vi "Idle_Insert.vi"(4 "Serial No":i32, 8 "error in (no error)":errorcluster, 11 "Ref in":T1={"MS SQL Connection"=refnum, "UDL File"=path "", "Time"="", "DCODE"="", "WIP+1"=0, "MC No?"=0, "POKAYOKE?"=FALSE, "Expected Result"="", "Result [Status]"="", "Clock"=0.0, "RFID"="", "WIP Queue"=refnum, "TS Parameter"={"ProfitCenterCode"="", "LineCode"="", "WorkOrderNumber"="", "Model"="", "Model_with_Prefix"="", "VendorCode"="", "SetParameterDateCode"="", "PokaYoke"=0, "Target"=1, "Live_DateCode"="", "CustomerPartNumber"="", "Hand"="", "sBarcode"=FALSE, "FCA"=0, "Ent_Stamp"=timestamp(0 s since 1904-01-01), "STS_CD"=0.0}, "Data_Queue"=[], "RFID Serial No."=""} {"TS Parameter"."FCA" format="%01d"; "TS Parameter"."Target" min=1 max=100000; "TS Parameter"."PokaYoke" min=0 max=1}) -> (0 "error out":errorcluster, 2 "Message":picture, 3 "Ref Out":T1={"MS SQL Connection"=refnum, "UDL File"=path "", "Time"="", "DCODE"="", "WIP+1"=0, "MC No?"=0, "POKAYOKE?"=FALSE, "Expected Result"="", "Result [Status]"="", "Clock"=0.0, "RFID"="", "WIP Queue"=refnum, "TS Parameter"={"ProfitCenterCode"="", "LineCode"="", "WorkOrderNumber"="", "Model"="", "Model_with_Prefix"="", "VendorCode"="", "SetParameterDateCode"="", "PokaYoke"=0, "Target"=1, "Live_DateCode"="", "CustomerPartNumber"="", "Hand"="", "sBarcode"=FALSE, "FCA"=0, "Ent_Stamp"=timestamp(0 s since 1904-01-01), "STS_CD"=0.0}, "Data_Queue"=[], "RFID Serial No."=""} {"TS Parameter"."FCA" format="%01d"; "TS Parameter"."Target" min=1 max=100000; "TS Parameter"."PokaYoke" min=0 max=1})   [LabVIEW 2020]
uses:
  Controls/TD SQL.ctl
  <vilib>/addons/database/Connection.llb/Conn ObjectReference.ctl
  Controls/WIP_State.ctl
  Controls/TS_Parameter.ctl
  Controls/Msg_Type.ctl
  MS SQL/MS_Global.vi
  <vilib>/addons/database/NI_Database_API.lvlib
panel:
  out "resulting string":string
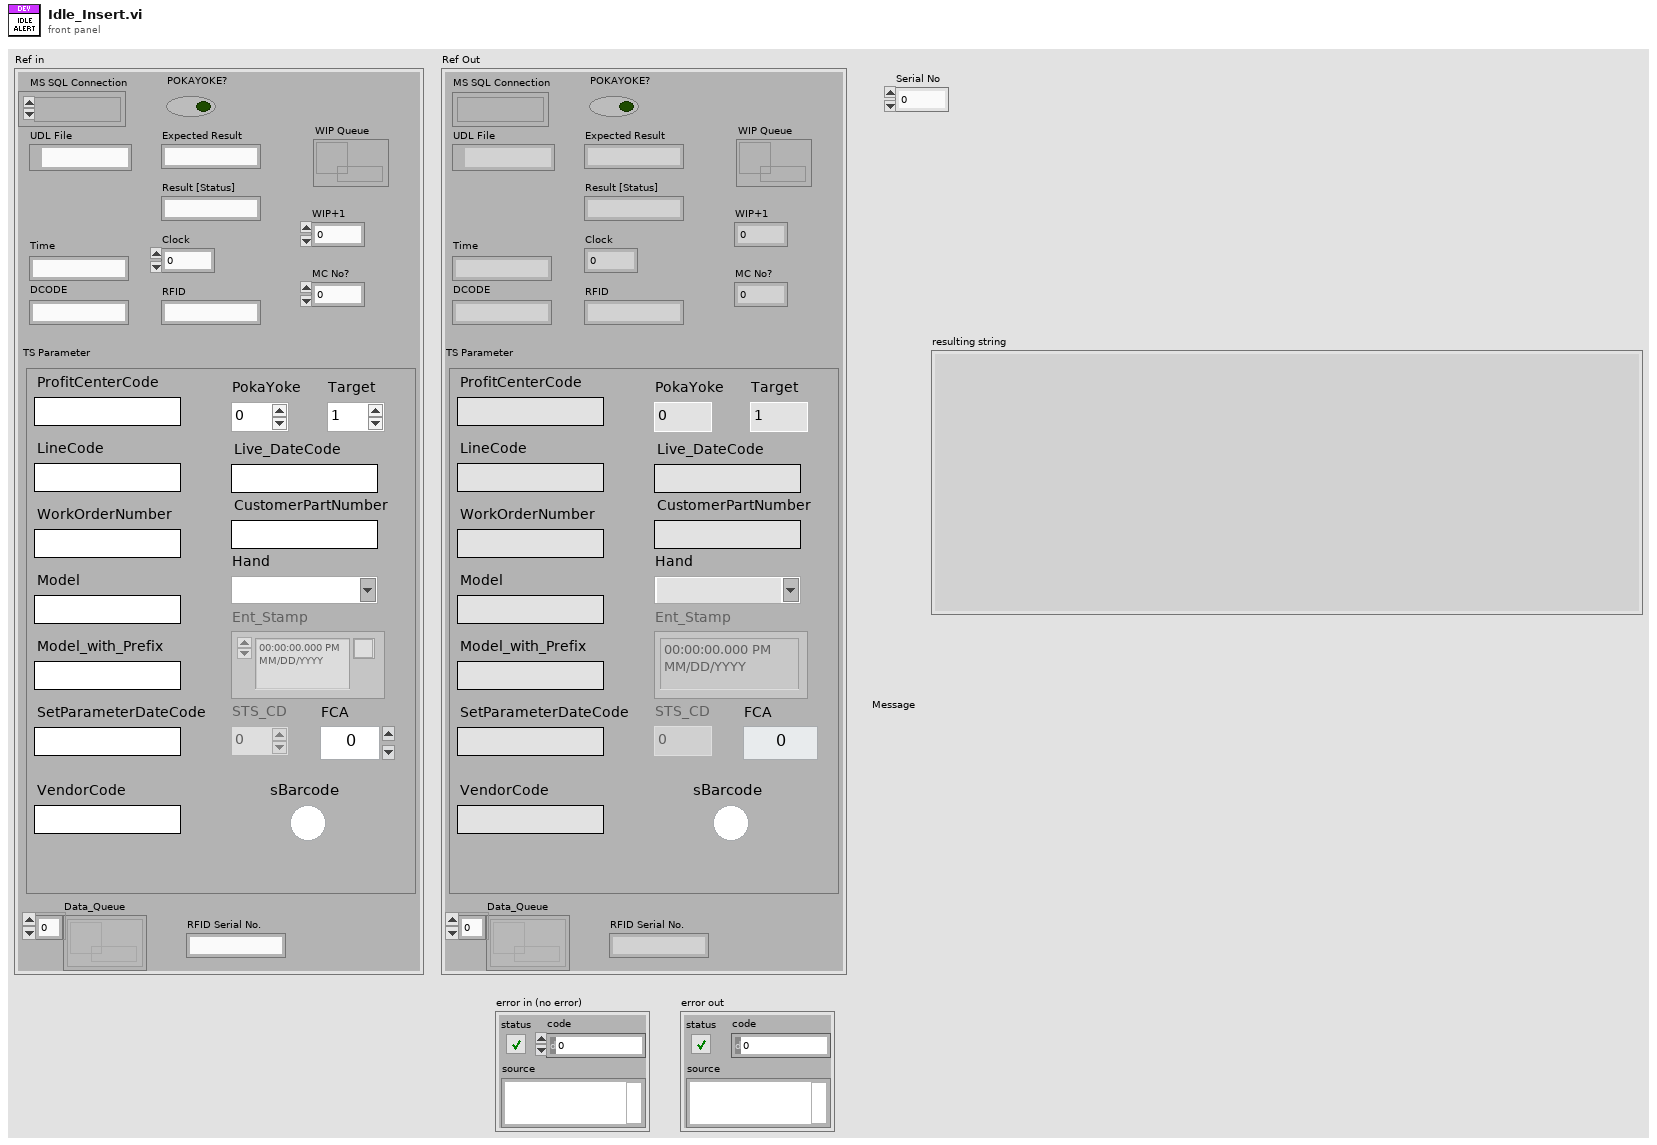
[diagram p1: front panel]
types:
  T1 = typedef "TD SQL.ctl" = cluster{"MS SQL Connection":T2, "UDL File":path, "Time":string, "DCODE":string, "WIP+1":i64, "MC No?":i32, "POKAYOKE?":bool, "Expected Result":string, "Result [Status]":string, "Clock":dbl, "RFID":string, "WIP Queue":refnum<queue>, "TS Parameter":T3, "Data_Queue":refnum<queue>[], "RFID Serial No.":string}
  T2 = typedef "NI_Database_API.lvlib/Conn ObjectReference.ctl" = refnum<k1>
  T3 = typedef "TS_Parameter.ctl" = cluster{"ProfitCenterCode":string, "LineCode":string, "WorkOrderNumber":string, "Model":string, "Model_with_Prefix":string, "VendorCode":string, "SetParameterDateCode":string, "PokaYoke":i32, "Target":i32, "Live_DateCode":string, "CustomerPartNumber":string, "Hand":string, "sBarcode":bool, "FCA":i32, "Ent_Stamp":timestamp, "STS_CD":dbl}
  T4 = typedef "Msg_Type.ctl" = enum16{"Normal", "Pass", "Fail", "Fault", "User", "Bypass", "Fail Save"}
  T5 = typedef "Idle_Timer.ctl" = cluster{"OP10":T6, "OP20":T6, "OP30":T6, "OP40":T6, "OP50":T6, "OP60":T6}
  T6 = typedef "Idle_Timer_disp.ctl" = dbl
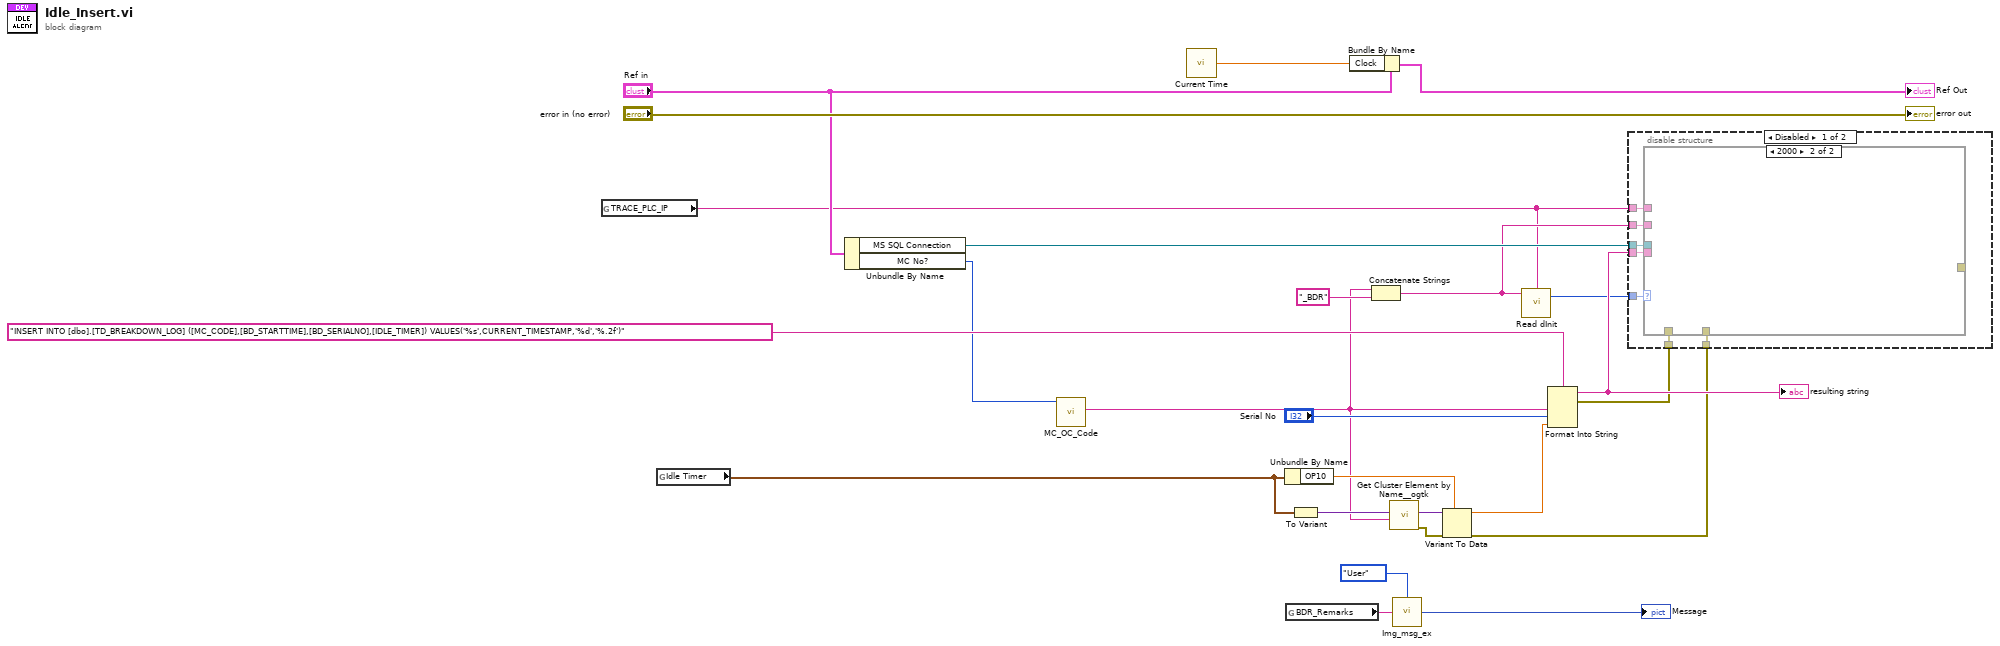
[diagram p0: block diagram]
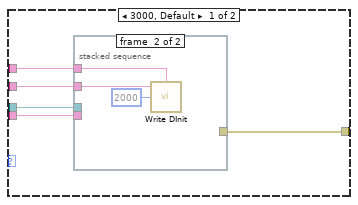
[diagram p2: hidden frame]
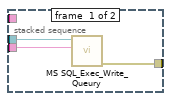
[diagram p3: hidden frame]
diagram:
  n1 = global read "MS_Global.vi" "TRACE_PLC_IP"() -> (w8:string)
  n2 = global read "MS_Global.vi" "Idle Timer"() -> (w15:T5)
  n3 = Unbundle By Name("Ref in") -> ("MS SQL Connection"=w23:T2, "MC No?"=w7:i32)
  n4 = call "MC_OC_Code.vi"("index"=w7) -> ("Machine Code"=w6:string)  [unwired: 4 in, 6 out]
  n5 = call <userlib>:"Current Time.vi"() -> ("Current Time (Sec)"=w1:dbl)  [unwired: 15 in]
  n6 = Unbundle By Name(w15) -> ("OP10"=w11:T6)
  n7 = global read "MS_Global.vi" "BDR_Remarks"() -> (w4:string)
  n8 = To Variant(anything=w15) -> (Variant=w14:variant)
  n9 = Bundle By Name(cluster="Ref in", "Clock"=w1) -> (→"Ref Out":T1)
  n10 = Concatenate Strings(w6, "_BDR" ("String")) -> (w18:string)
  n11 = call <userlib>:"Get Cluster Element by Name__ogtk.vi"("Element Name"=w6, "Cluster"=w14) -> ("error out"=w12:errorcluster, "VElement"=w13:variant)  [unwired: 7 in, 1 out]
  n12 = call "Img_msg_ex.vi"("Msg Type"=Msg_Type."User", "Message In"=w4) -> ("Message"=→"Message":picture)  [unwired: 2 in]
  n13 = Variant To Data(error in=w12, type=w11, Variant=w13) -> (data=w10:T6, error out=w9:errorcluster)
  n14 = call "Read dInit.vi"("Network Path"=w8, "Tag Name"=w18) -> ("Numeric"=w19:i32)  [unwired: 3 in]
  n15 = Format Into String(format string="INSERT INTO [dbo].[TD_BREAKDOWN_LOG] ([MC_CODE],[BD_STARTTIME],[BD_SERIALNO],[IDLE_TIMER]) VALUES('%s',CURRENT_TIMESTAMP,'%d','%.2f')" ("Query"), w6, "Serial No", w10) -> (resulting string=w21:string, error out=w17:errorcluster)  [unwired: 2 in]
  "resulting string" <- w21
  n16 = disable-structure shown="Disabled" {
    disable-tunnel: w23 -> [w32 _]
    disable-tunnel: w21 -> [w31 _]
    disable-tunnel: w19 -> [w30 _]
    disable-tunnel: w18 -> [w29 _]
    disable-tunnel: w8 -> [w28 _]
    disable-tunnel: w17 -> [w27 _]
    disable-tunnel: w9 -> [w26 _]
    frame Disabled {
      n17 = case shown="2000" w30 {
        tunnel: w32 -> [w37 _]
        tunnel: w31 -> [w36 _]
        tunnel: [w35 _] -> _
        tunnel: w28 -> [w34 _]
        tunnel: w29 -> [w33 _]
        tunnel: w27 -> [_ _]
        tunnel: w26 -> [_ _]
        frame 3000, Default {
          n18 = stacked-sequence {
            tunnel: w37 -> [w40 _]
            tunnel: w36 -> [w39 _]
            tunnel: [w38 _] -> w35
            tunnel: w34 -> [_ w42]
            tunnel: w33 -> [_ w41]
            frame #0 {
              n19 = call "MS SQL_Exec_Write_Queury.vi"("Query"=w39, "Refnum in"=w40) -> ("error out"=w38:errorcluster)  [unwired: 8 in, 1 out]
            }
            frame #1 {
              n20 = call "Write DInit.vi"("Network Path"=w42, "Int"=2000, "Tag Name"=w41) -> ()  [unwired: 2 in]
            }
          }
        }
        frame 2000 {
        }
      }
    }
    frame Enabled {
    }
  }
  "error out" <- "error in (no error)"
